vi "Echosounder.vi"() -> ()   [LabVIEW 2014]
uses:
  <vilib>/Analysis/NI_AALPro.lvlib
panel:
  in  "停止":bool
  out "回声探测":dbl[](graph)
  out "回声信号":dbl[](graph)
  in  "回声延时":i32(slide)=50 scale=0.0..250.0
  in  "频率":dbl(slide)=20.0 scale=0.0..50.0
  in  "衰减值":dbl(slide)=100.0 scale=0.0..200.0
  in  "采样数":i32=500
  in  "回声振幅":dbl(slide)=0.1 scale=0.0..0.5 scale format="%.2g"
  # "回声探测器"
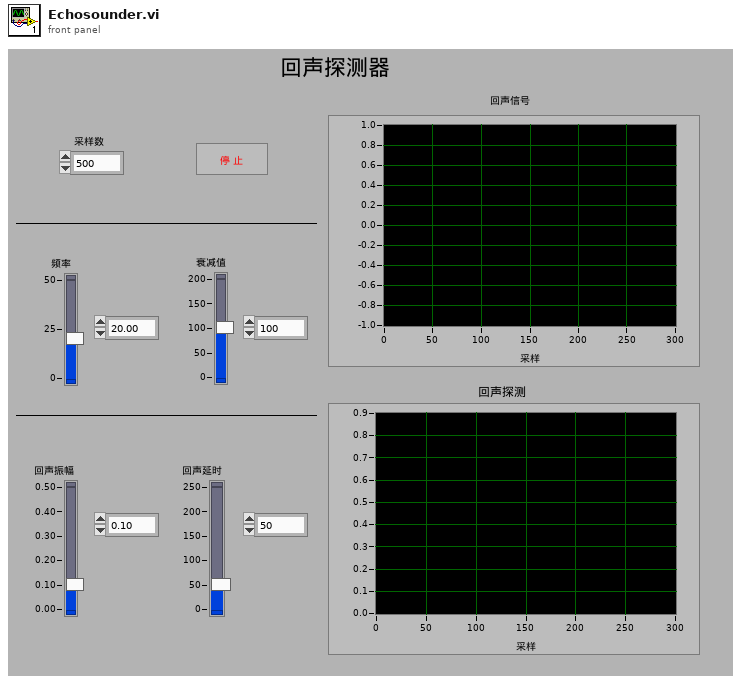
[diagram p1: front panel]
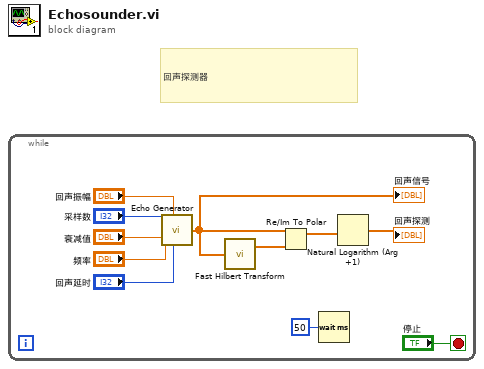
[diagram p0: block diagram]
diagram:
  # "回声探测器"
  n1 = while {
    stop <- "停止" stop-if-true
    n2 = call "Echo Generator.vi"("回声延时"="回声延时", "回声振幅"="回声振幅", "频率"="频率", "衰减值"="衰减值", "采样数"="采样数") -> ("回声信号"=w5:dbl[])  [unwired: 1 in]
    "回声信号" <- w5
    n3 = call <vilib>:"Fast Hilbert Transform.vi"("X"=w5) -> ("Hilbert{X}"=w4:dbl[])  [unwired: 1 out]
    n4 = Re/Im To Polar(2:w4, 3:w5) -> (1:w3:dbl[])  [unwired: 1 out]
    n5 = Wait (ms)(milliseconds to wait=u32 50 ("等待时间（毫秒）")) -> ()  [unwired: 1 out]
    n6 = Natural Logarithm (Arg +1)(1:w3) -> (0:→"回声探测":dbl[])
  }
